vi "MATLAB - Lorenz Diff Eq.vi"() -> ()   [LabVIEW 2023]
doc: "Demonstrates how to call into MATLAB(R) code using the MATLAB nodes. This VI solves a Lorenz Attractor differential equation and plots the resulting Lorenz Attractor. The MATLAB(R) Application Software release R2016a or later must be installed in order to run this VI."
uses:
  <vilib>/Math Plots/3D Math Plots/3D Comet/3D Comet XCtrl/3D Comet.xctl
  <vilib>/Math Plots/3D Math Plots/3D Comet/3D Comet Datatype/Public/Plot Helper (Vector).vi
  <vilib>/Math Plots/3D Math Plots/3D Comet/3D Comet Datatype/3D Comet Datatype.lvclass
panel:
  out "3D Comet":refnum<class "3D Plot Datatype.lvclass">[](xcontrol)
  out "Lorenz Attractor":cluster{"t":dbl[], "Y":dbl[]}[](graph)
  # "Overview: Solves a Lorenz Attractor differential equation using the MATLAB node and plots the resulting Lorenz Attractor.\nRequirements: LabVIEW Full Development System, MATLAB(R) Application Software release R2016a or later.\nInstructions: Run the VI."
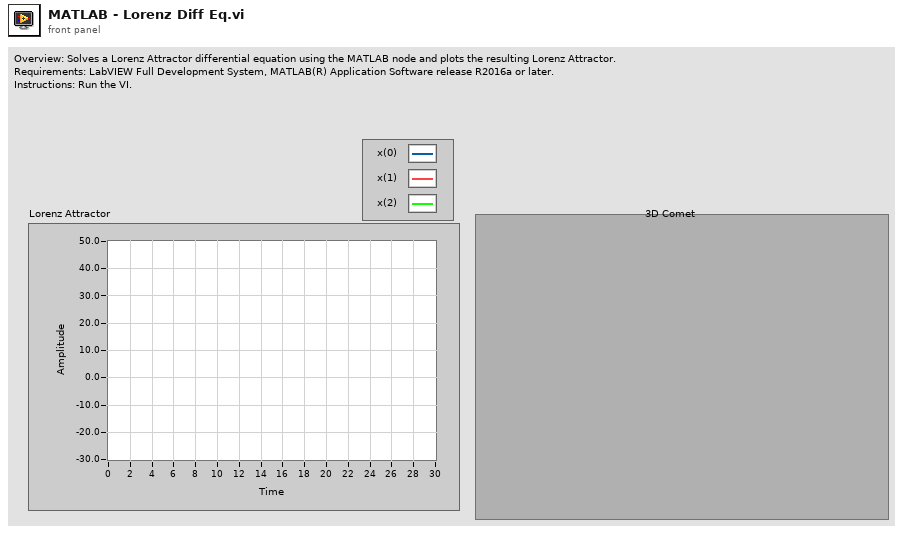
[diagram p1: front panel]
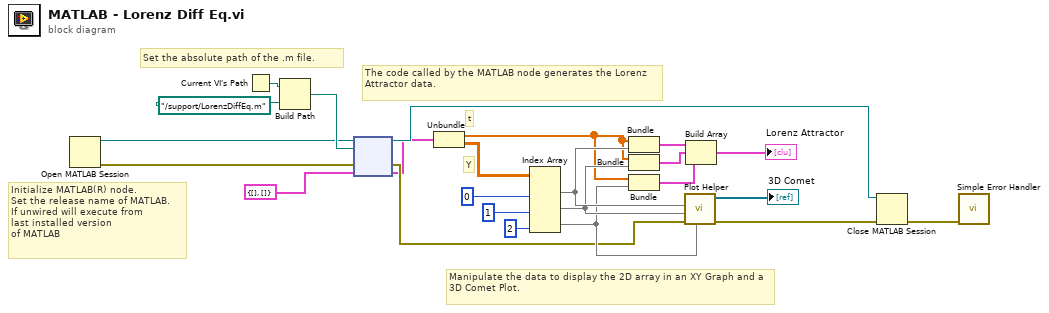
[diagram p0: block diagram]
diagram:
  # "t"
  # "Set the absolute path of the .m file."
  # "Y"
  # "Initialize MATLAB(R) node.\nSet the release name of MATLAB.\nIf unwired will execute from \nlast installed version \nof MATLAB"
  # "Manipulate the data to display the 2D array in an XY Graph and a 3D Comet Plot."
  # "The code called by the MATLAB node generates the Lorenz Attractor data."
  n1 = Open MATLAB Session() -> (8:w10:refnum<k37>, 11:w9:errorcluster)  [unwired: 2 in]
  n2 = Current VI's Path() -> (path=w8:path)
  n3 = Build Path(base path=w8, name or relative path=path "../support/LorenzDiffEq.m") -> (appended path=w11:path)
  n4 = node(w10, w11, w9, cluster{"Element1":dbl[], "Element2":dbl[][]} {"Element1"=[], "Element2"=[]}) -> (w13:refnum<k37>, w7:errorcluster, w5:cluster{"Element1":dbl[], "Element2":dbl[][]})  [unwired: 1 in, 2 out]
  n5 = Unbundle(w5) -> ("Element1"=w3:dbl[], "Element2"=w4:dbl[][])
  n6 = Index Array(array=w4, index (col) #1=0 ("disabled index (col)"), index (col) #2=1 ("index (col)"), index (col) #3=2 ("index (col)")) -> (element #1=w20:dbl[], element #2=w18:dbl[], element #3=w16:dbl[])  [unwired: 3 in]
  n7 = Bundle("Element1"=w3, "Element2"=w20) -> (w19:cluster{"Element1":dbl[], "Element2":dbl[]})  [unwired: 1 in]
  n8 = Bundle("Element1"=w3, "Element2"=w18) -> (w17:cluster{"Element1":dbl[], "Element2":dbl[]})  [unwired: 1 in]
  n9 = Bundle("Element1"=w3, "Element2"=w16) -> (w15:cluster{"Element1":dbl[], "Element2":dbl[]})  [unwired: 1 in]
  n10 = call-poly <vilib>:"Plot Helper.vi"("z vector"=w16, "error in (no error)"=w7, "y vector"=w18, "x vector"=w20) -> ("error out"=w2:errorcluster, "3D Plot lvclass Array out"=→"3D Comet":refnum<class "3D Plot Datatype.lvclass">[])  [unwired: 2 in, 4 out]
  n11 = Build Array(w19, w17, w15) -> (→"Lorenz Attractor":cluster{"Element1":dbl[], "Element2":dbl[]}[])
  n12 = Close MATLAB Session(0:w13, 3:w2) -> (11:w1:errorcluster)
  n13 = call <vilib>:"Simple Error Handler.vi"("error in (no error)"=w1) -> ()  [unwired: 4 in, 5 out]
